vi "String to csv.vi"(0 "Sorted array":string[](array[string]), 11 "error in":errorcluster) -> (15 "error out":errorcluster)   [LabVIEW 2020, in "Custom Sort Function.lvlib"]
doc: "This VI is used to stored the sorted data in the form of csv"
uses:
  Custom Sort Function.lvlib
panel:
  out "Description":string
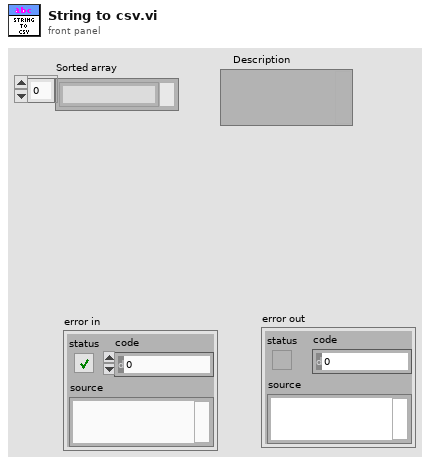
[diagram p1: front panel]
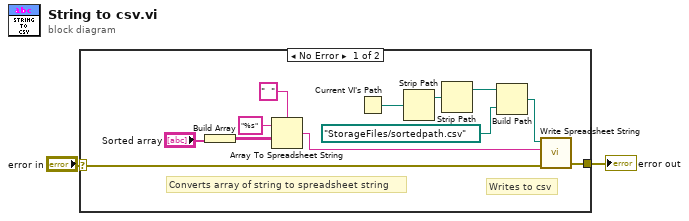
[diagram p0: block diagram]
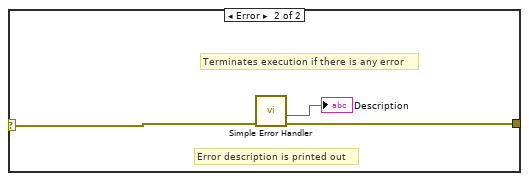
[diagram p2: hidden frame]
diagram:
  n1 = case shown="No Error" "error in" {
    selector: "error in" -> [w4 w17]
    tunnel: [w12 w16] -> w2
    frame No Error {
      # "Writes to csv"
      # "Converts array of string to spreadsheet string"
      n2 = Build Array("Sorted array") -> (w13:string[][])
      n3 = Array To Spreadsheet String(delimiter (Tab)="  ", array=w13, 3:"%s" ("format string")) -> (spreadsheet string=w11:string)
      n4 = Current VI's Path() -> (path=w10:path)
      n5 = Strip Path(path=w10) -> (stripped path=w9:path)  [unwired: 1 out]
      n6 = Strip Path(path=w9) -> (stripped path=w7:path)  [unwired: 1 out]
      n7 = Build Path(base path=w7, name or relative path=path "StorageFiles/sortedpath.csv") -> (appended path=w6:path)
      n8 = call <vilib>:"Write Spreadsheet String.vi"("error in"=w4, "spreadsheet string"=w11, "file path (dialog if empty)"=w6) -> ("error out"=w12:errorcluster)  [unwired: 7 in, 1 out]
    }
    frame Error {
      # "Error description is printed out"
      # "Terminates execution if there is any error"
      n9 = call <vilib>:"Simple Error Handler.vi"("error in (no error)"=w17) -> ("source out"=→"Description":string, "error out"=w16:errorcluster)  [unwired: 4 in, 3 out]
    }
  }
  "error out" <- w2
